vi "CoordinateTransform_CreateMatrix.vi"(2 "error in (no error)":errorcluster, 3 "Input CCD, Galvo -Reference":T1(array[cluster])=[{"CCDx"=0.0, "CCDy"=0.0, "GalvoX"=3.0, "GalvoY"=4.0}, {"CCDx"=0.0, "CCDy"=100.0, "GalvoX"=3.0, "GalvoY"=8.0}, {"CCDx"=100.0, "CCDy"=0.0, "GalvoX"=6.0, "GalvoY"=4.0}]) -> (0 "error out":errorcluster, 1 "Conversion Matrix":dbl[][](array[numeric]))   [LabVIEW 2011]
uses:
  <vilib>/Analysis/7linalg.llb/Solve Linear Equations (single right hand).vi
  <vilib>/Analysis/7linalg.llb/Solve Linear Eqs (General).vi
  <vilib>/Analysis/7linalg.llb/Solve Linear Eqs (Gen, single right hand).vi
  <vilib>/Analysis/NI_AALPro.lvlib
panel:
  # "old! new: calibration_createMatrix with array input"
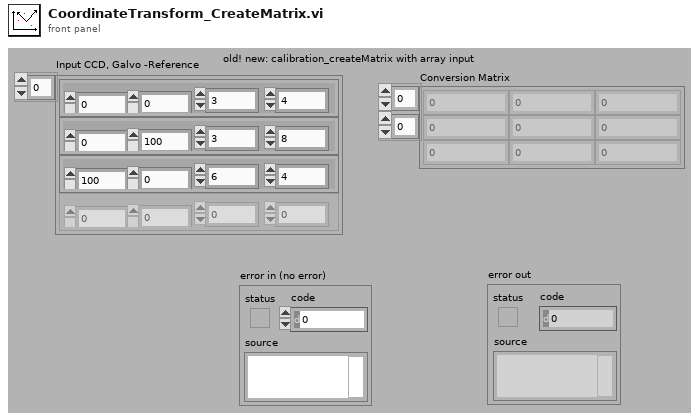
[diagram p1: front panel]
types:
  T1 = cluster{"CCDx":dbl, "CCDy":dbl, "GalvoX":dbl, "GalvoY":dbl}[]
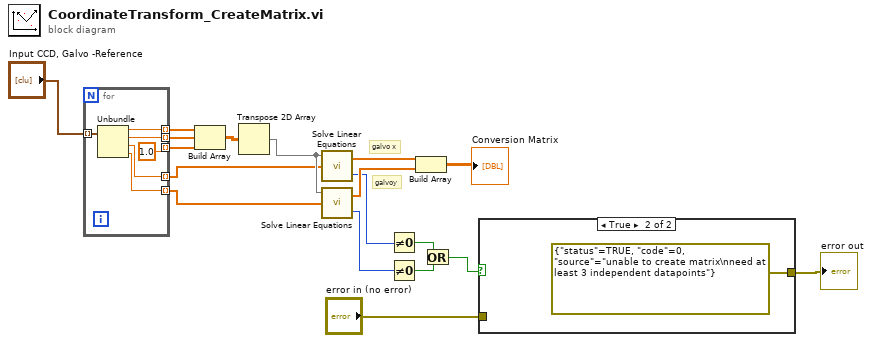
[diagram p0: block diagram]
diagram:
  # "galvoy"
  # "galvo x"
  n1 = for {
    tunnel: "Input CCD, Galvo -Reference" -> [w24] mode=indexing
    tunnel: [w23] -> w14 mode=indexing
    tunnel: [w22] -> w13 mode=indexing
    tunnel: [1.0] -> w12 mode=indexing
    tunnel: [w20] -> w9 mode=indexing
    tunnel: [w19] -> w8 mode=indexing
    n2 = Unbundle(w24) -> ("CCDx"=w23:dbl, "CCDy"=w22:dbl, "GalvoX"=w20:dbl, "GalvoY"=w19:dbl)
  }
  n3 = Build Array(w14, w13, w12) -> (w17:dbl[][])
  n4 = Transpose 2D Array(2D array=w17) -> (transposed array=w11:dbl[][])
  n5 = call-poly <vilib>:"Solve Linear Equations.vi"("Known Vector"=w9, "Input Matrix"=w11) -> ("error"=w7:i32, "Solution Vector"=w16:dbl[])  [unwired: 1 in]
  n6 = call-poly <vilib>:"Solve Linear Equations.vi"("Known Vector"=w8, "Input Matrix"=w11) -> ("error"=w6:i32, "Solution Vector"=w15:dbl[])  [unwired: 1 in]
  n7 = Not Equal To 0?(x=w7) -> (x != 0?=w5:bool)
  n8 = Not Equal To 0?(x=w6) -> (x != 0?=w4:bool)
  n9 = Build Array(w16, w15) -> (→"Conversion Matrix":dbl[][])
  n10 = Or(x=w5, y=w4) -> (x .or. y?=w3:bool)
  n11 = case shown="True" w3 {
    tunnel: "error in (no error)" -> [w25 _]
    tunnel: [w25 errorcluster {"status"=TRUE, "code"=0, "source"="unable to create matrix\nneed at least 3 independent datapoints"} ("error in (no error)")] -> w1
    frame False {
    }
    frame True {
    }
  }
  "error out" <- w1
